vi "Data_Analysis_Global_var.vi"() -> ()   [LabVIEW 2019]
panel:
  in  "group names array":string[][](array[string])
  in  "FileArray":string[](array[string])
  in  "tdms file out":refnum<k34>
  in  "TDMS array":refnum<k34>[](array[refnum])
  in  "group names":string[](array[string])
  in  "Listbox":i32[](array[numeric])
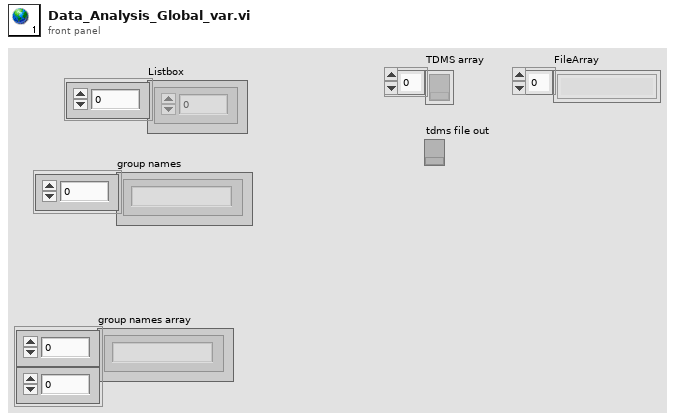
[diagram p1: front panel]
diagram:
